vi "Remote SLB.vi"(8 "Command":string, 9 "Init":bool, 10 "Slave to Master File":path, 11 "Master to Slave File":path) -> (1 "Message\nBack":string, 2 "Failed":bool, 3 "Success":bool)   [LabVIEW 2014]
uses:
  Rem Master Case.ctl
panel:
  out "Read Error":errorcluster
  out "Write Error":errorcluster
  # "Remote SLB VI"
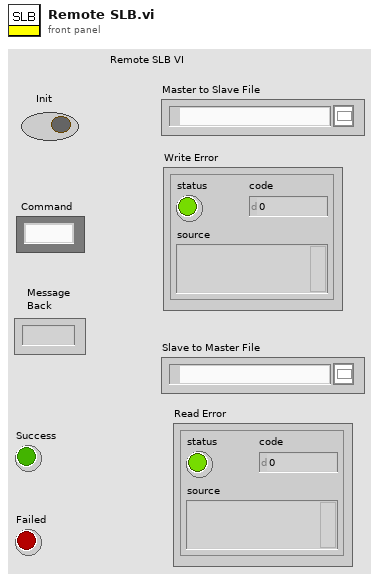
[diagram p1: front panel]
types:
  T1 = typedef "Rem Master Case.ctl" = enum16{"init", "send command", "wait for HS = 1", "send HS = 0", "wait for HS = 0", "end success", "end failure"}
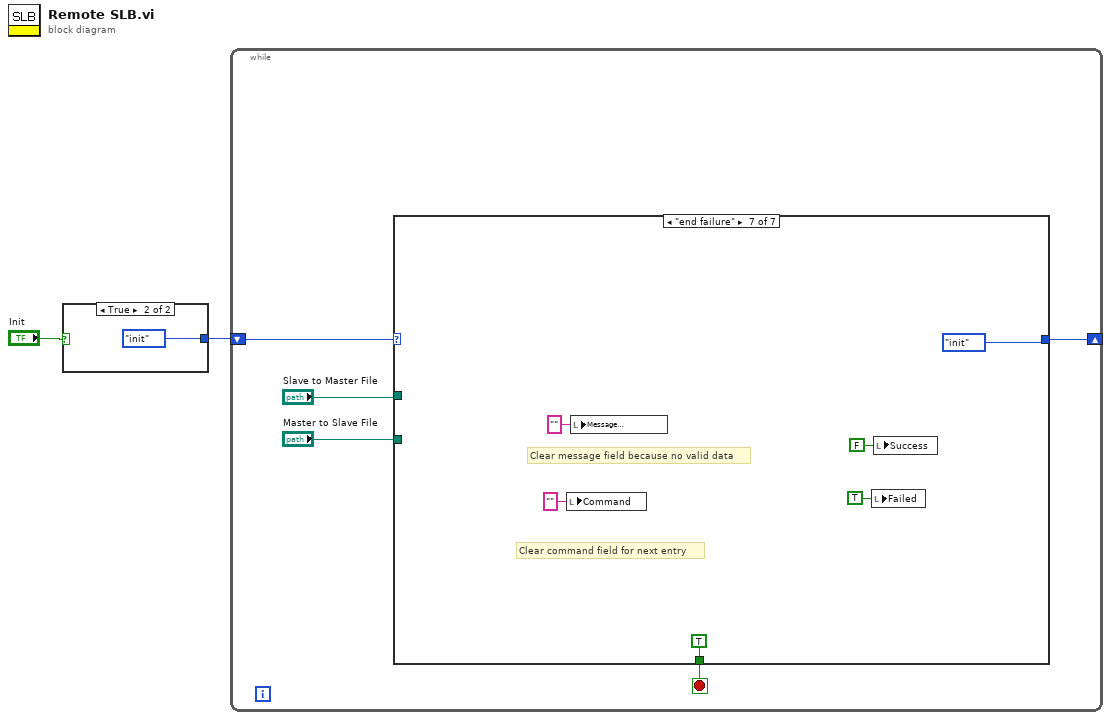
[diagram p0: block diagram]
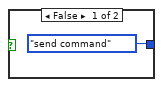
[diagram p2: hidden frame]
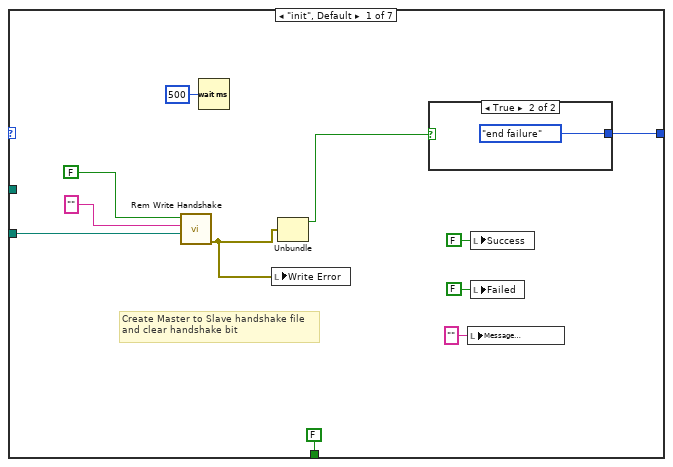
[diagram p3: hidden frame]
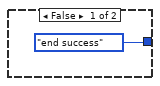
[diagram p4: hidden frame]
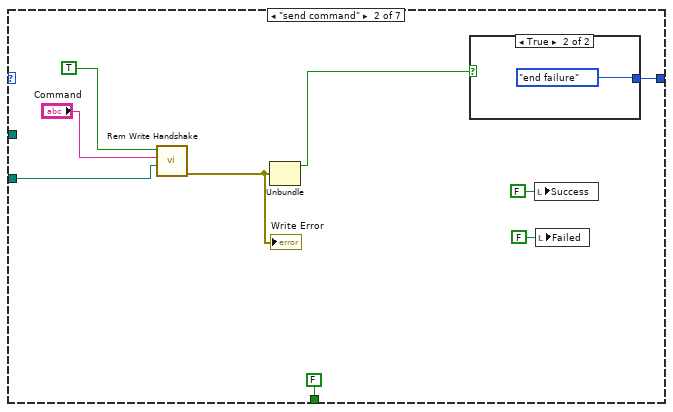
[diagram p5: hidden frame]
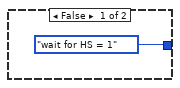
[diagram p6: hidden frame]
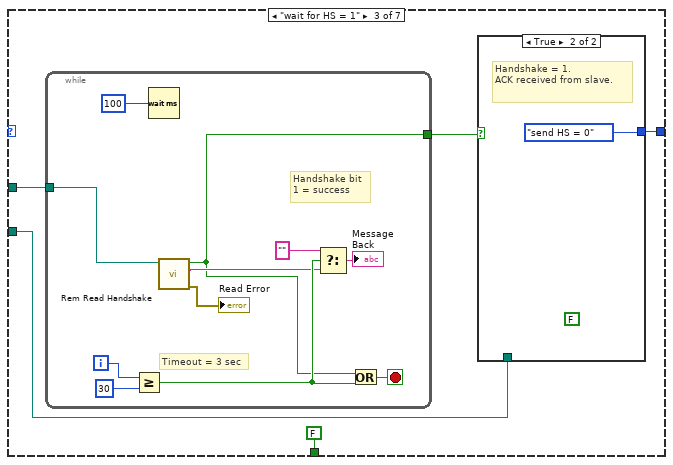
[diagram p7: hidden frame]
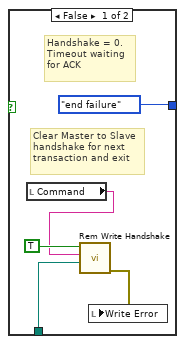
[diagram p8: hidden frame]
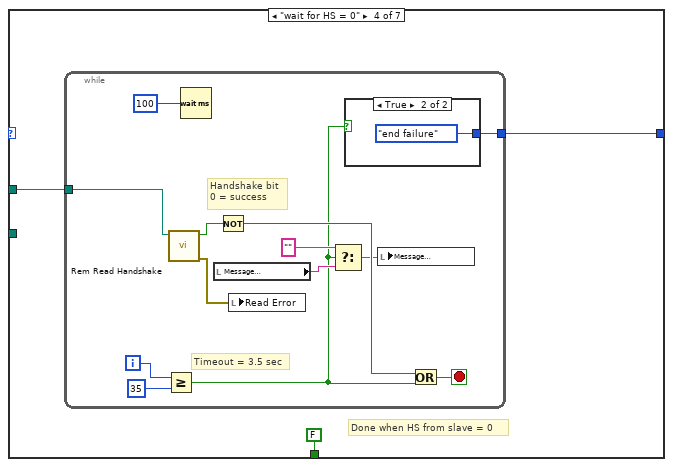
[diagram p9: hidden frame]
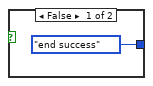
[diagram p10: hidden frame]
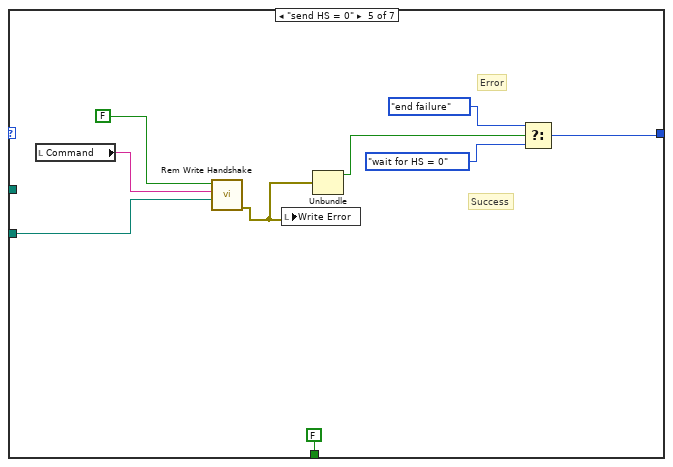
[diagram p11: hidden frame]
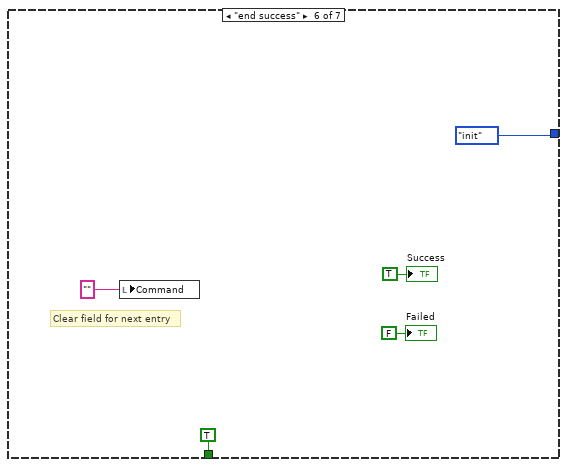
[diagram p12: hidden frame]
diagram:
  n1 = case shown="True" "Init" {
    tunnel: [Rem_Master_Case."send command" ("Enum") Rem_Master_Case."init" ("Enum")] -> w1
    frame False {
    }
    frame True {
    }
  }
  n2 = while {
    shift-right: [w8] -> _
    shift-left: w1 -> [w7]
    stop <- w9 stop-if-true
    n3 = case shown="\"end failure\"" w7 {
      tunnel: [FALSE ("Stop Button") FALSE ("Stop Button") FALSE ("status") FALSE ("Stop Button") FALSE ("Stop Button") TRUE ("Stop Button") TRUE ("Stop Button")] -> w9
      tunnel: [w20 w31 w36 w56 w82 Rem_Master_Case."init" ("Enum") Rem_Master_Case."init" ("Enum")] -> w8
      tunnel: "Slave to Master File" -> [_ _ w38 w58 _ _ _]
      tunnel: "Master to Slave File" -> [w14 w27 w37 _ w79 _ _]
      frame "init", Default {
        # "Create Master to Slave handshake file\nand clear handshake bit"
        n4 = call "Rem Write Handshake.vi"("Handshake"=FALSE, "String In"="", "File Path Control"=w14) -> ("error out"=w11:errorcluster)  [unwired: 7 in]
        n5 = Wait (ms)(milliseconds to wait=u32 500) -> ()  [unwired: 1 out]
        n6 = local write "Write Error"(w11) -> ()
        n7 = Unbundle(w11) -> ("status"=w10:bool)  [unwired: 2 out]
        n8 = case shown="True" w10 {
          tunnel: [Rem_Master_Case."end success" ("Enum") Rem_Master_Case."end failure" ("Enum")] -> w20
          frame False {
          }
          frame True {
          }
        }
        n9 = local write "Message\nBack"("" ("Received Char")) -> ()
        n10 = local write "Success"(FALSE ("Success")) -> ()
        n11 = local write "Failed"(FALSE ("Failed")) -> ()
      }
      frame "send command" {
        n12 = call "Rem Write Handshake.vi"("Handshake"=TRUE, "String In"="Command", "File Path Control"=w27) -> ("error out"=w24:errorcluster)  [unwired: 7 in]
        "Write Error" <- w24
        n13 = Unbundle(w24) -> ("status"=w23:bool)  [unwired: 2 out]
        n14 = case shown="True" w23 {
          tunnel: [Rem_Master_Case."wait for HS = 1" ("Enum") Rem_Master_Case."end failure" ("Enum")] -> w31
          frame False {
          }
          frame True {
          }
        }
        n15 = local write "Success"(FALSE ("Success")) -> ()
        n16 = local write "Failed"(FALSE ("Failed")) -> ()
      }
      frame "wait for HS = 1" {
        n17 = while {
          tunnel: w38 -> [w48]
          tunnel: [w45] -> w35
          i -> [w51]
          stop <- w54 stop-if-true
          # "Handshake bit\n1 = success"
          # "Timeout = 3 sec"
          n18 = Greater Or Equal?(x=w51, y=30 ("x")) -> (x >= y?=w52:bool)
          n19 = Wait (ms)(milliseconds to wait=u32 100) -> ()  [unwired: 1 out]
          n20 = call "Rem Read Handshake.vi"("File Path Control"=w48) -> ("error out"=→"Read Error":errorcluster, "string after HS bit"=w46:string, "HS bit = 1"=w45:bool)  [unwired: 8 in]
          n21 = Select(t="", s=w52, f=w46) -> (s? t:f=→"Message\nBack":string)
          n22 = Or(x=w45, y=w52) -> (x .or. y?=w54:bool)
        }
        n23 = case shown="True" w35 {
          tunnel: w37 -> [w42 _]
          tunnel: [Rem_Master_Case."end failure" ("Enum") Rem_Master_Case."send HS = 0" ("Enum")] -> w36
          frame False {
            # "Clear Master to Slave\nhandshake for next\ntransaction and exit"
            # "Handshake = 0.\nTimeout waiting\nfor ACK"
            n24 = local read "Command"() -> (w41:string)
            n25 = call "Rem Write Handshake.vi"("Handshake"=TRUE, "String In"=w41, "File Path Control"=w42) -> ("error out"=w40:errorcluster)  [unwired: 7 in]
            n26 = local write "Write Error"(w40) -> ()
          }
          frame True {
            (unwired) FALSE ("Stop Button")
            # "Handshake = 1.\nACK received from slave."
          }
        }
      }
      frame "wait for HS = 0" {
        # "Done when HS from slave = 0"
        n27 = while {
          tunnel: w58 -> [w61]
          tunnel: [w62] -> w56
          i -> [w68]
          stop <- w70 stop-if-true
          # "Handshake bit\n0 = success"
          # "Timeout = 3.5 sec"
          n28 = Greater Or Equal?(x=w68, y=35 ("x")) -> (x >= y?=w63:bool)
          n29 = call "Rem Read Handshake.vi"("File Path Control"=w61) -> ("error out"=w59:errorcluster, "HS bit = 1"=w60:bool)  [unwired: 8 in, 1 out]
          n30 = Wait (ms)(milliseconds to wait=u32 100) -> ()  [unwired: 1 out]
          n31 = local read "Message\nBack"() -> (w65:string)
          n32 = Not(x=w60) -> (.not. x?=w66:bool)
          n33 = local write "Read Error"(w59) -> ()
          n34 = Select(t="", s=w63, f=w65) -> (s? t:f=w64:string)
          n35 = case shown="True" w63 {
            tunnel: [Rem_Master_Case."end success" ("Enum") Rem_Master_Case."end failure" ("Enum")] -> w62
            frame False {
            }
            frame True {
            }
          }
          n36 = local write "Message\nBack"(w64) -> ()
          n37 = Or(x=w66, y=w63) -> (x .or. y?=w70:bool)
        }
      }
      frame "send HS = 0" {
        # "Success"
        # "Error"
        n38 = local read "Command"() -> (w76:string)
        n39 = call "Rem Write Handshake.vi"("Handshake"=FALSE, "String In"=w76, "File Path Control"=w79) -> ("error out"=w77:errorcluster)  [unwired: 7 in]
        n40 = local write "Write Error"(w77) -> ()
        n41 = Unbundle(w77) -> ("status"=w81:bool)  [unwired: 2 out]
        n42 = Select(t=Rem_Master_Case."end failure" ("Enum"), s=w81, f=Rem_Master_Case."wait for HS = 0" ("Enum")) -> (s? t:f=w82:T1)
      }
      frame "end success" {
        # "Clear field for next entry"
        n43 = local write "Command"("" ("Message\nOut")) -> ()
        "Failed" <- FALSE ("Failed")
        "Success" <- TRUE ("Success")
      }
      frame "end failure" {
        # "Clear message field because no valid data"
        # "Clear command field for next entry"
        n44 = local write "Command"("" ("Command")) -> ()
        n45 = local write "Message\nBack"("" ("Message\nBack")) -> ()
        n46 = local write "Failed"(TRUE ("Failed")) -> ()
        n47 = local write "Success"(FALSE ("Success")) -> ()
      }
    }
  }
